vi "thermal_optical_camera_V2.vi"() -> ()   [LabVIEW 2025]
uses:
  <vilib>/vision/driver/NI_Vision_Acquisition_Software.lvlib
panel:
  in  "millisecond timer value":u32
  in  "File Path":string="C:\\Digambar\\Metal_thin_wall\\Optical_images\\Optical_images"
  in  "Stop (F)":bool
  in  "Acquisition Control:\nExposure Time [100, 3E7]":dbl=999.0 caption="Acquisition Control::Exposure Time" min=100.0 max=29999995.0
  in  "Analog Control:\nGain [0, 27]":dbl caption="Analog Control::Gain" min=0.0 max=27.045663671679687
  in  "Analog Control:\nBlack Level [-5, 10]":dbl caption="Analog Control::Black Level" min=-5.0000011920928955 max=10.000002384185791
  in  "Analog Control:\nGamma [0.25, 4.00]":dbl=0.800048828125 caption="Analog Control::Gamma" min=0.25 max=4.0 step=0.05
  out "Optical camera":T1(plugin-control)
  in  "capture interval (s) for optical camera":dbl
  out "Camera Information Array":T2(array[cluster]) {"BusType" format="%x"; "SerialNumberLow" format="%.0x"; "SerialNumberHigh" format="%.0x"}
  in  "Connected Only? (Yes)":bool=TRUE
  in  "capture interval (s) for thermal camera":dbl
  out "Thermal camera":T1(plugin-control)
  out "IP address":string
  out "Output":string
  in  "Flag":bool
  in  "Stop recording":bool
  in  "Stop Preview":bool
  in  "Focus":dbl(slide) scale=0.0..100.0
  in  "Record":bool
  out "?":string
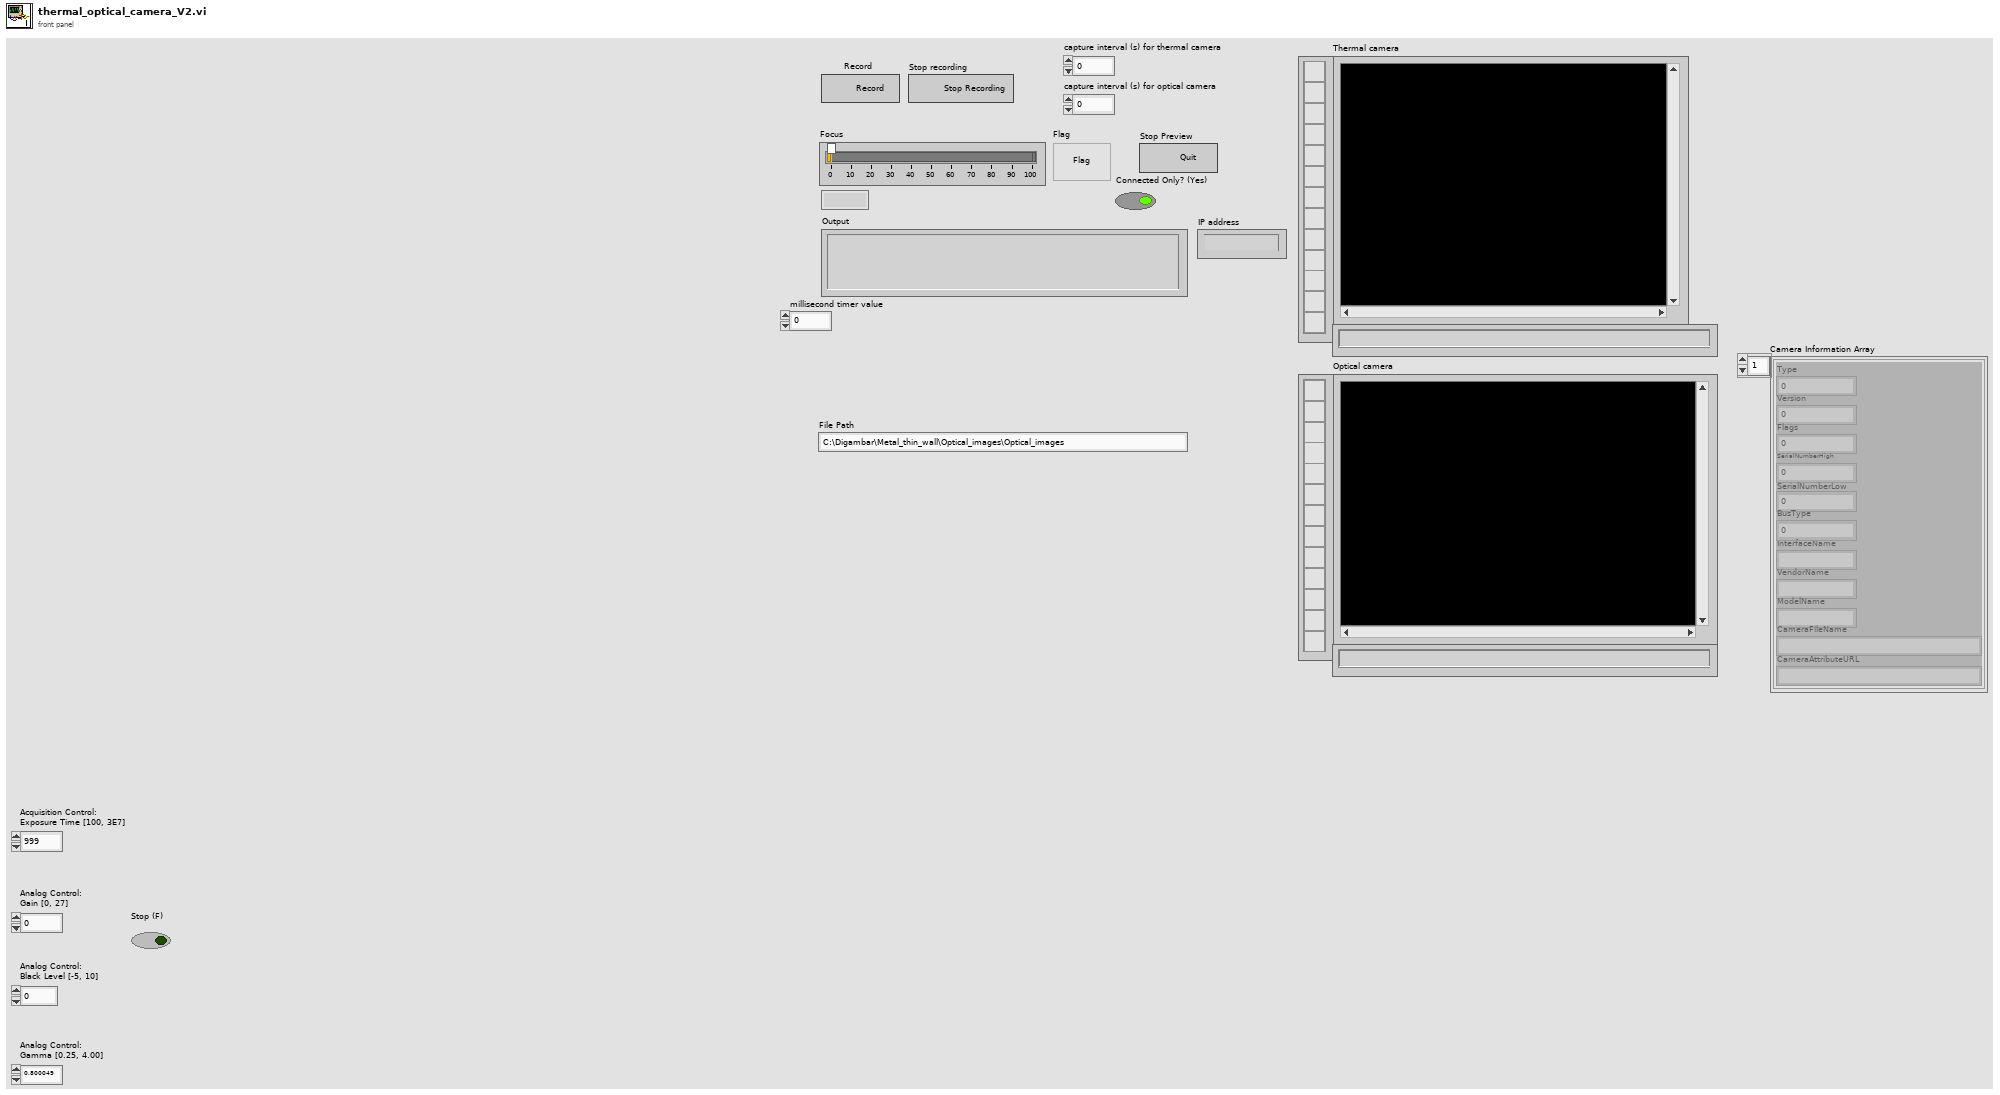
[diagram p1: front panel]
types:
  T1 = typedef "IMAQ Image.ctl" = refnum<image>
  T2 = cluster{"Type":u32, "Version":u32, "Flags":u32, "SerialNumberHigh":u32, "SerialNumberLow":u32, "BusType":u32, "InterfaceName":string, "VendorName":string, "ModelName":string, "CameraFileName":string, "CameraAttributeURL":string}[]
  T3 = enum16{"open", "replace", "create", "open or create", "replace or create", "replace or create with confirmation"}
  T4 = enum16{"big-endian, network order", "native, host order", "little-endian"}
  T5 = enum16{"Standard", "Buffered", "CRLF", "Immediate"}
  T6 = typedef "Image Type" = u32
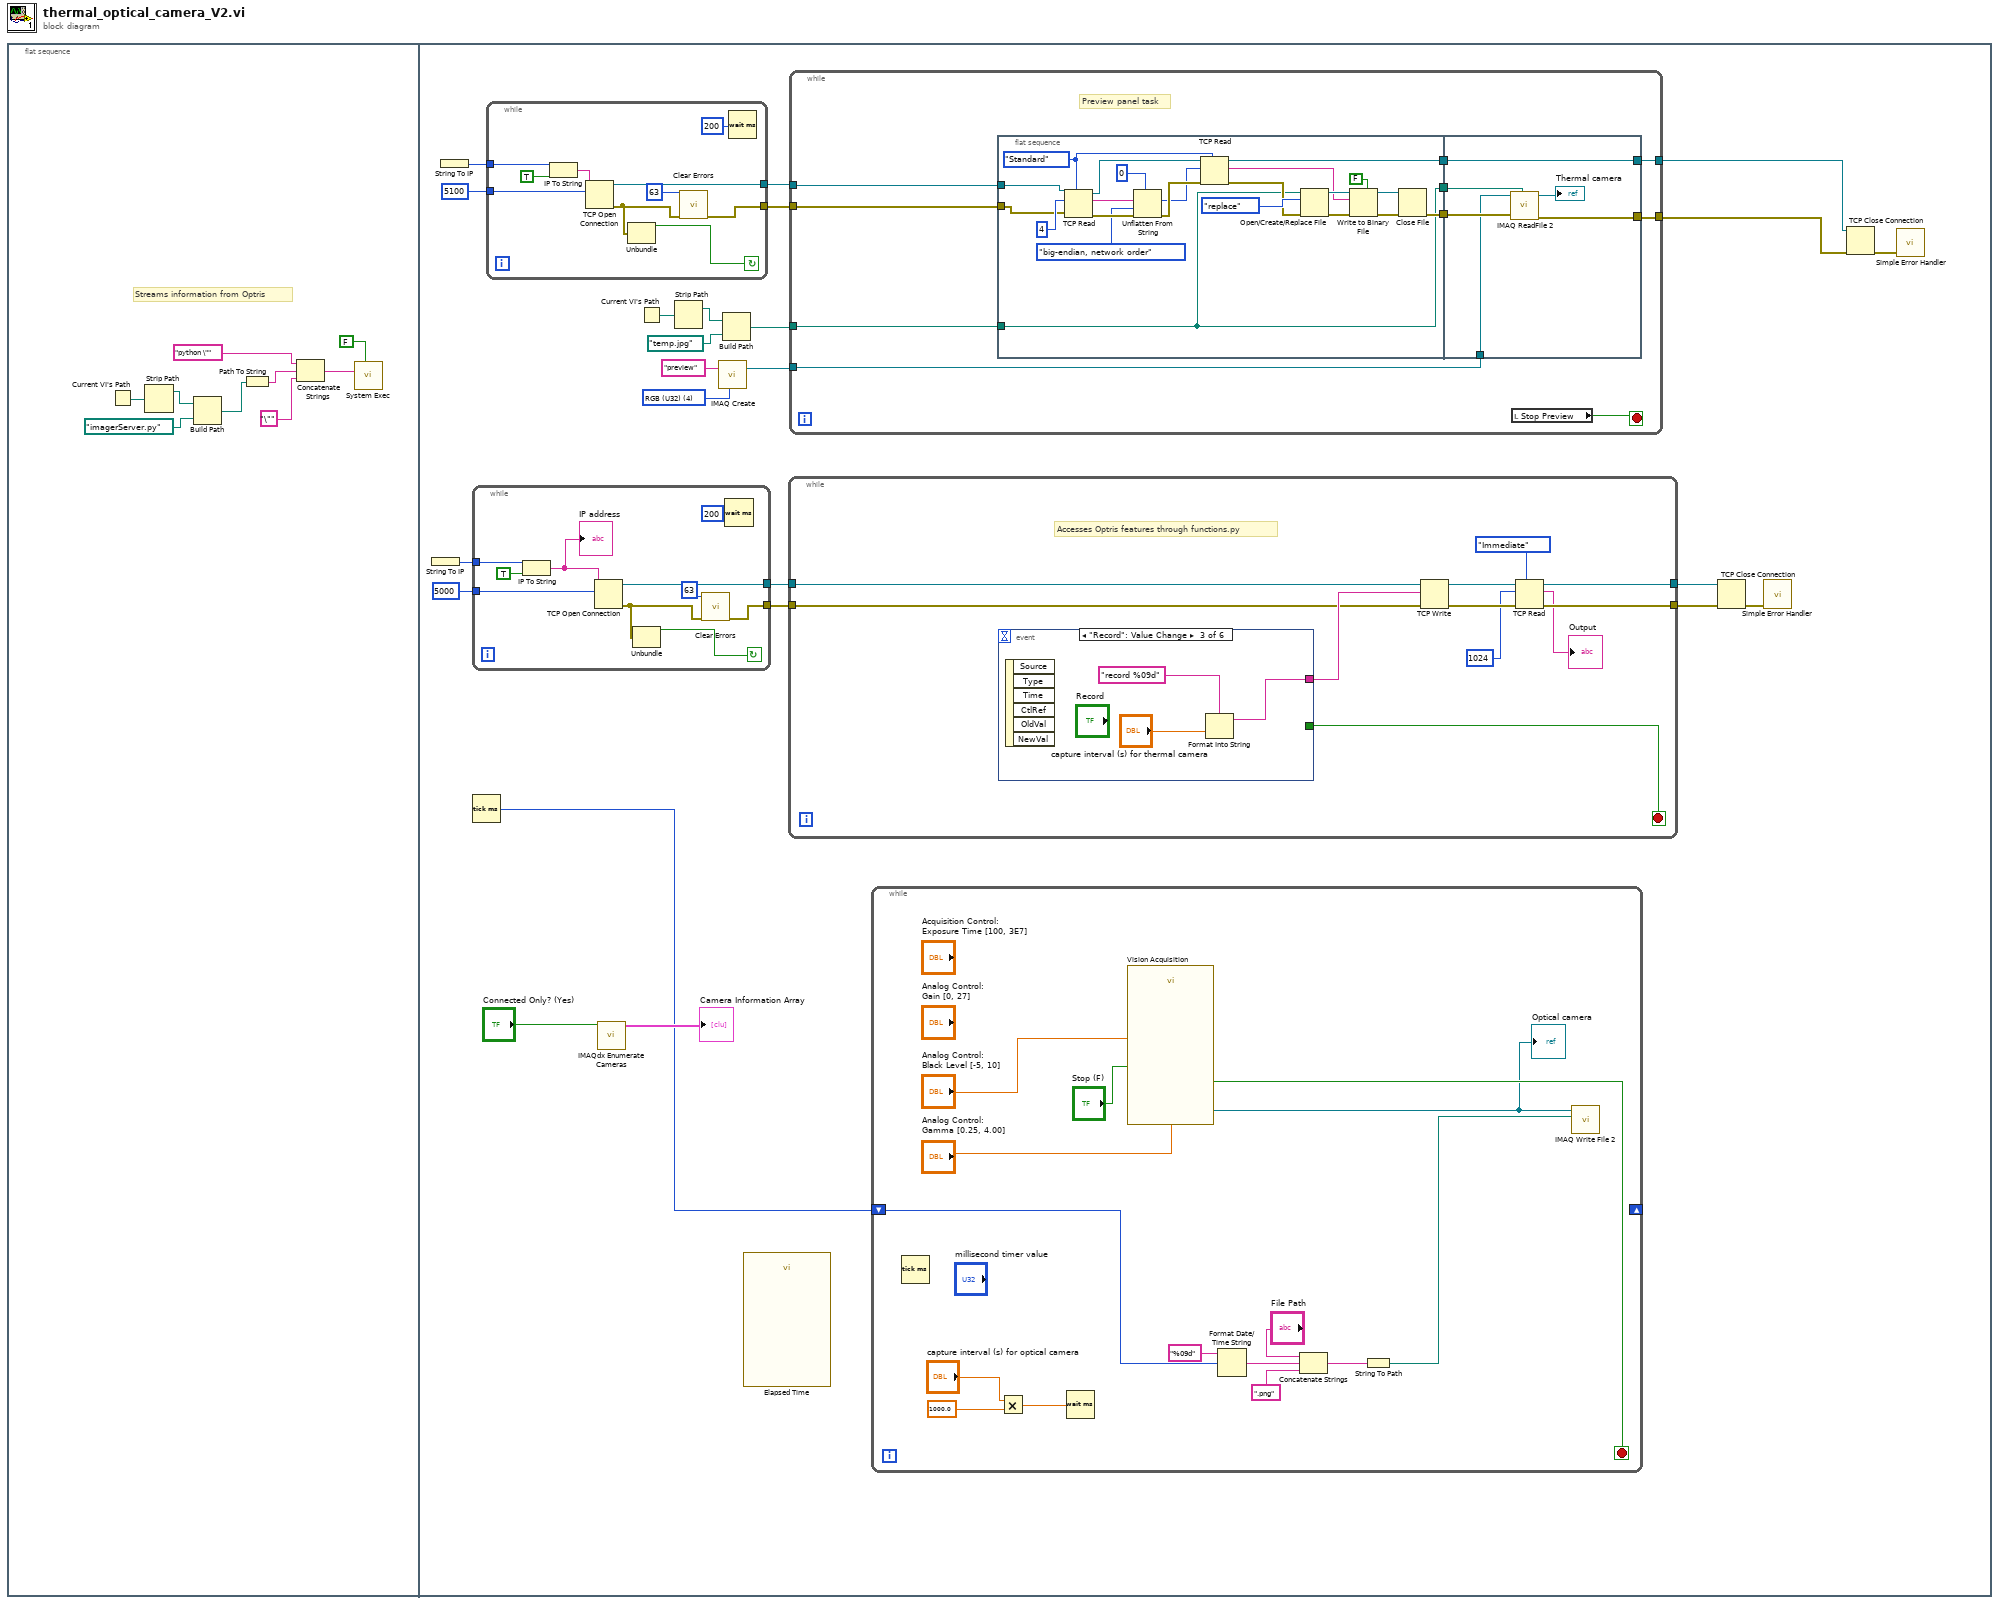
[diagram p0: block diagram]
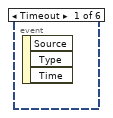
[diagram p2: hidden frame]
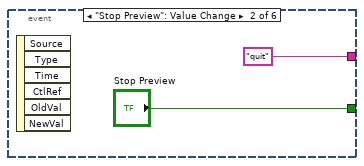
[diagram p3: hidden frame]
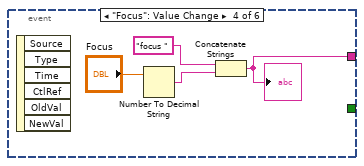
[diagram p4: hidden frame]
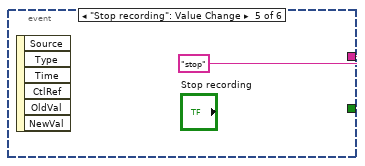
[diagram p5: hidden frame]
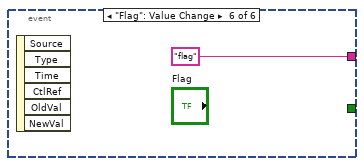
[diagram p6: hidden frame]
diagram:
  n1 = flat-sequence {
    frame #0 {
      # "Streams information from Optris"
      n2 = Current VI's Path() -> (path=w4:path)
      n3 = Strip Path(path=w4) -> (stripped path=w5:path)  [unwired: 1 out]
      n4 = Build Path(base path=w5, name or relative path=path "imagerServer.py") -> (appended path=w2:path)
      n5 = Path To String(path=w2) -> (string=w8:string)
      n6 = Concatenate Strings("python \"" ("string"), w8, "\"" ("string")) -> (w7:string)
      n7 = call <vilib>:"System Exec.vi"("wait until completion? (T)"=FALSE, "command line"=w7) -> ()  [unwired: 6 in, 4 out]
    }
    frame #1 {
      w21 = T6 4 items=["Grayscale (U8)", "Grayscale (I16)", "Grayscale (SGL)", "Complex (CSG)", "RGB (U32)", "HSL (U32)", "RGB (U64)", "Grayscale (U16)"] ("Image Type")
      n8 = String To IP() -> (0:w18:u32)  [unwired: 1 in]
      n9 = String To IP() -> (0:w16:u32)  [unwired: 1 in]
      n10 = while {
        tunnel: [w62] -> w20
        tunnel: [w68] -> w19
        tunnel: w18 -> [w66]
        tunnel: u16 5000 ("remote port or service name") -> [w64]
        stop <- w59 continue-if-true
        n11 = IP To String(1:TRUE ("dot notation? (F)"), 2:w66) -> (0:w67:string)
        "IP address" <- w67
        n12 = TCP Open Connection(address=w67, remote port or service name=w64) -> (connection ID=w68:refnum<k5>, error out=w63:errorcluster)  [unwired: 3 in]
        n13 = Unbundle(w63) -> ("status"=w59:bool)  [unwired: 2 out]
        n14 = call <vilib>:"Clear Errors.vi"("error in (no error)"=w63, "specific error code to clear (0: all)"=63) -> ("error out"=w62:errorcluster)  [unwired: 4 in, 1 out]
        n15 = Wait (ms)(milliseconds to wait=u32 200) -> ()  [unwired: 1 out]
      }
      n16 = Tick Count (ms)() -> (millisecond timer value=w10:u32)
      n17 = while {
        tunnel: w16 -> [w58]
        tunnel: [w52] -> w15
        tunnel: [w56] -> w14
        tunnel: u16 5100 ("remote port or service name") -> [w54]
        stop <- w49 continue-if-true
        n18 = IP To String(1:TRUE ("dot notation? (F)"), 2:w58) -> (0:w57:string)
        n19 = TCP Open Connection(address=w57, remote port or service name=w54) -> (connection ID=w56:refnum<k5>, error out=w53:errorcluster)  [unwired: 3 in]
        n20 = Unbundle(w53) -> ("status"=w49:bool)  [unwired: 2 out]
        n21 = call <vilib>:"Clear Errors.vi"("error in (no error)"=w53, "specific error code to clear (0: all)"=63) -> ("error out"=w52:errorcluster)  [unwired: 4 in, 1 out]
        n22 = Wait (ms)(milliseconds to wait=u32 200) -> ()  [unwired: 1 out]
      }
      n23 = call <vilib>:"IMAQdx Enumerate Cameras.vi"("Connected Only? (Yes)"="Connected Only? (Yes)") -> ("Camera Information Array"=→"Camera Information Array":T2)  [unwired: 9 in, 1 out]
      n24 = Current VI's Path() -> (path=w32:path)
      n25 = Strip Path(path=w32) -> (stripped path=w33:path)  [unwired: 1 out]
      n26 = call "IMAQ Create"("Image Name"="preview", "Image Type"=w21) -> ("New Image"=w28:T1)  [unwired: 3 in, 1 out]
      n27 = Build Path(base path=w33, name or relative path=path "temp.jpg") -> (appended path=w31:path)
      n28 = call "Elapsed Time"() -> ()  [unwired: 12 in, 8 out]
      n29 = while {
        tunnel: [w116] -> w24
        tunnel: [w114] -> w25
        tunnel: w20 -> [w112]
        tunnel: w19 -> [w111]
        stop <- w107 stop-if-true
        # "Accesses Optris features through functions.py"
        n30 = event shown="[2] \"Record\": Value Change" {
          selector: _ -> [_ _ _ _ _ _]
          dyn-events: _ -> [_ _ _ _ _ _]
          timeout: _ -> [_ _ _ _ _ _]
          tunnel: [_ "quit" w122 w124 "stop" "flag"] -> w113
          tunnel: [_ "Stop Preview" _ _ _ _] -> w107
          event Timeout {
            n31 = event-data() -> ()  [unwired: 1 in, 3 out]
          }
          event "Stop Preview": Value Change {
            n32 = event-data() -> ()  [unwired: 1 in, 6 out]
          }
          event "Record": Value Change {
            n33 = event-data() -> ()  [unwired: 1 in, 6 out]
            n34 = Format Into String(format string="record %09d", "capture interval (s) for thermal camera") -> (resulting string=w122:string)  [unwired: 2 in, 1 out]
          }
          event "Focus": Value Change {
            n35 = event-data() -> ()  [unwired: 1 in, 6 out]
            n36 = Number To Decimal String(number="Focus") -> (decimal integer string=w126:string)  [unwired: 1 in]
            n37 = Concatenate Strings("focus ", w126) -> (w124:string)
            "?" <- w124
          }
          event "Stop recording": Value Change {
            n38 = event-data() -> ()  [unwired: 1 in, 6 out]
          }
          event "Flag": Value Change {
            n39 = event-data() -> ()  [unwired: 1 in, 6 out]
          }
        }
        n40 = TCP Write(connection ID=w111, data in=w113, error in (no error)=w112) -> (connection ID out=w115:refnum<k5>, error out=w117:errorcluster)  [unwired: 1 in, 1 out]
        n41 = TCP Read(connection ID=w115, bytes to read=1024, error in (no error)=w117, 7:T5."Immediate" ("mode (standard)")) -> (connection ID out=w114:refnum<k5>, data out=→"Output":string, error out=w116:errorcluster)  [unwired: 1 in]
      }
      n42 = while {
        tunnel: w28 -> [w73]
        tunnel: [w74] -> w29
        tunnel: [w78] -> w30
        tunnel: w31 -> [w76]
        tunnel: w15 -> [w71]
        tunnel: w14 -> [w70]
        stop <- w69 stop-if-true
        # "Preview panel task"
        n43 = flat-sequence {
          tunnel: w76 -> [w82]
          tunnel: [w84] -> w77
          tunnel: [w83] -> w75
          tunnel: [w82] -> w72
          tunnel: w71 -> [w80]
          tunnel: w70 -> [w79]
          tunnel: [w106] -> w78
          tunnel: w77 -> [w106]
          tunnel: w75 -> [w105]
          tunnel: [w104] -> w74
          tunnel: w73 -> [w103]
          tunnel: w72 -> [w102]
          frame #0 {
            w93 = T5."Standard" ("mode (standard)")
            n44 = TCP Read(connection ID=w79, bytes to read=4, error in (no error)=w80, 7:w93) -> (connection ID out=w96:refnum<k5>, data out=w81:string, error out=w99:errorcluster)  [unwired: 1 in]
            n45 = Unflatten From String(type=0, binary string=w81, byte order (0:big-endian, network order)=T4."big-endian, network order", error in (no error)=w99) -> (value=w94:i32, error out=w95:errorcluster)  [unwired: 1 in, 1 out]
            n46 = TCP Read(connection ID=w96, bytes to read=w94, error in (no error)=w95, 7:w93) -> (connection ID out=w84:refnum<k5>, data out=w89:string, error out=w91:errorcluster)  [unwired: 1 in]
            n47 = Open/Create/Replace File(file path (use dialog)=w82, error in=w91, operation (0:open)=T3."replace") -> (refnum out=w90:refnum<file>, error out=w87:errorcluster)  [unwired: 3 in, 1 out]
            n48 = Write to Binary File(file (use dialog)=w90, data=w89, error in=w87, 5:FALSE ("prepend array or string size? (T)")) -> (refnum out=w85:refnum<file>, error out=w86:errorcluster)  [unwired: 2 in, 1 out]
            n49 = Close File(refnum=w85, error in=w86) -> (error out=w83:errorcluster)  [unwired: 1 out]
          }
          frame #1 {
            n50 = call "IMAQ ReadFile 2"("File Path"=w102, "error in (no error)"=w105, "Image"=w103) -> ("error out"=w104:errorcluster, "Image Out"=→"Thermal camera":T1)  [unwired: 4 in, 3 out]
          }
        }
        n51 = local read "Stop Preview"() -> (w69:bool)
      }
      n52 = while {
        shift-right: _ -> [_]
        shift-left: w10 -> [w35]
        stop <- w47 stop-if-true
        n53 = Tick Count (ms)() -> ()  [unwired: 1 out]
        n54 = Multiply(x="capture interval (s) for optical camera", y=1000.0) -> (x*y=w40:dbl)
        n55 = Wait (ms)(milliseconds to wait=w40) -> ()  [unwired: 1 out]
        n56 = call "Vision Acquisition"("Analog Control::Black Level"="Analog Control:\nBlack Level [-5, 10]", "Analog Control::Gamma"="Analog Control:\nGamma [0.25, 4.00]", "Stop (F)"="Stop (F)") -> ("Image Out"=w46:T1, "Stopped"=w47:bool)  [unwired: 22 in, 1 out]
        "Optical camera" <- w46
        n57 = Format Date/Time String(time format string (%c)="%09d", seconds (now)=w35) -> (date/time string=w36:string)  [unwired: 1 in]
        n58 = Concatenate Strings("File Path", w36, ".png" ("string")) -> (w43:string)
        n59 = String To Path(string=w43) -> (path=w38:path)
        n60 = call-poly "IMAQ Write File 2"("File Path"=w38, "Image"=w46) -> ()  [unwired: 8 in, 2 out]
      }
      n61 = TCP Close Connection(connection ID=w25, error in (no error)=w24) -> (error out=w26:errorcluster)  [unwired: 1 in, 1 out]
      n62 = call <vilib>:"Simple Error Handler.vi"("error in (no error)"=w26) -> ()  [unwired: 4 in, 5 out]
      n63 = TCP Close Connection(connection ID=w30, error in (no error)=w29) -> (error out=w27:errorcluster)  [unwired: 1 in, 1 out]
      n64 = call <vilib>:"Simple Error Handler.vi"("error in (no error)"=w27) -> ()  [unwired: 4 in, 5 out]
    }
  }
